vi "Open TCP Session.vi"(7 "Slave ID (255)":u8=255, 8 "error in (no error)":errorcluster, 9 "Timeout (10000)":i32=10000, 10 "Port (502)":u16=502, 11 "IP Address":string="localhost") -> (0 "error out":errorcluster, 3 "MB_TCP session":refnum<class "MB_Master_TCP.lvclass">)   [LabVIEW 2016, in "MB Master.lvlib" / "MB_Master_TCP.lvclass"]
doc: "Opens a new modbus session and establish the TCP connection. Note that the slave ID is set to the default of 0xFF. Slave ID can be changed later via the property node \"Slave ID\"."
uses:
  MB_Master_TCP.lvclass
  MB_ADU/MB_ADU.lvclass/MB_ADU.ctl
  MB_ADU_TCP/MB_ADU_TCP.lvclass/MB_ADU_TCP.ctl
  MB_Master_TCP.lvclass/MB_Master_TCP.ctl
  MB_ADU/Build ADU.vi
  MB_ADU_TCP/MB_ADU_TCP.lvclass
  C:/Users/PRANAV/Downloads/Modbus-Master-master (7)/Modbus-Master-master/MB_ADU/MB_ADU.lvclass
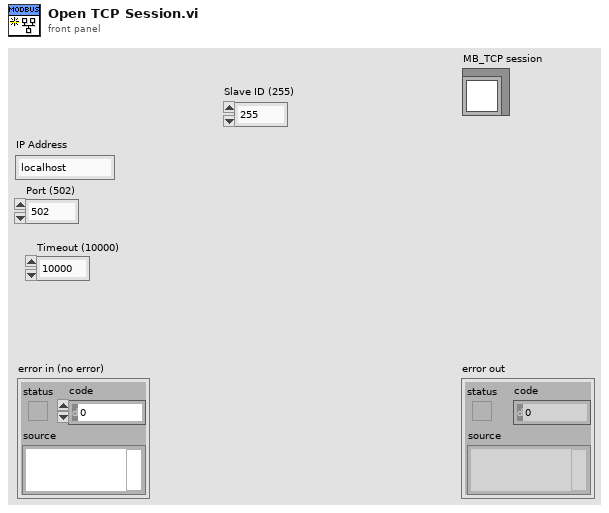
[diagram p1: front panel]
types:
  T1 = cluster{"IP Address":string, "Port":u16, "Timeout":i32, "Notifier":refnum<notifier>}
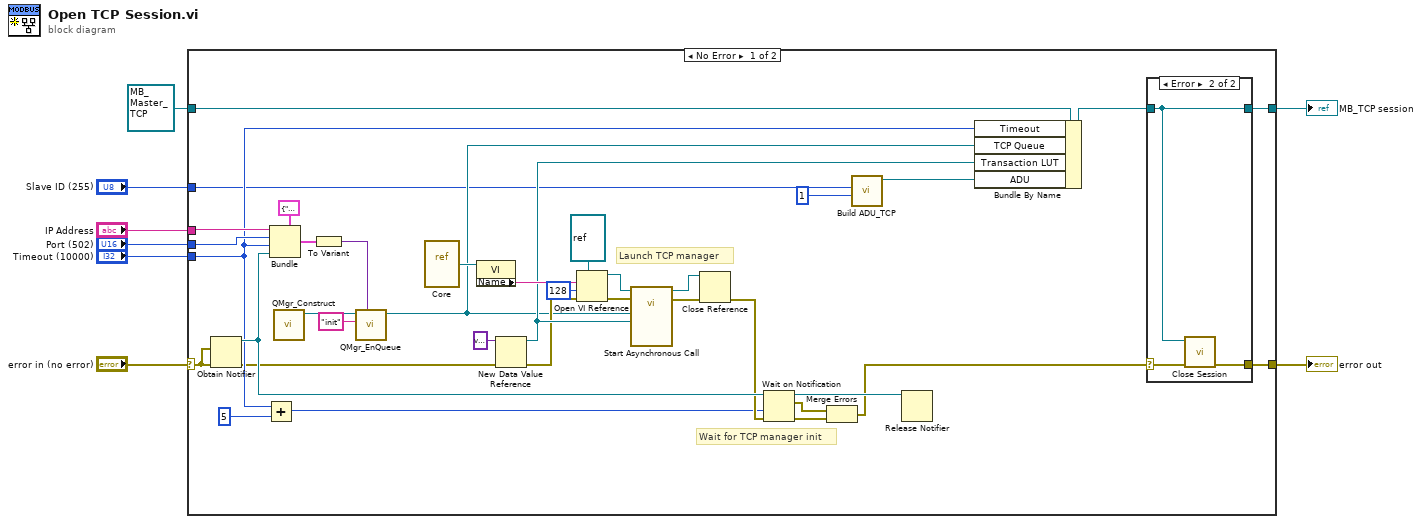
[diagram p0: block diagram]
diagram:
  n1 = case shown="No Error" "error in (no error)" {
    selector: "error in (no error)" -> [w22 w52]
    tunnel: [w26 w52] -> w7
    tunnel: [w28 w51] -> w5
    tunnel: refnum<class "MB_Master_TCP.lvclass"> refnum ("MB_Master_TCP in") -> [w45 w51]
    tunnel: "IP Address" -> [w41 _]
    tunnel: "Port (502)" -> [w40 _]
    tunnel: "Timeout (10000)" -> [w18 _]
    tunnel: "Slave ID (255)" -> [w9 _]
    frame No Error {
      # "Wait for TCP manager init"
      # "Launch TCP manager"
      n2 = Obtain Notifier(notification data type=w22, error in (no error)=w22) -> (notifier out=w31:refnum<notifier>, error out=w10:errorcluster)  [unwired: 2 in, 1 out]
      n3 = Add(x=w18, y=5) -> (x+y=w16:i32)
      n4 = Bundle(cluster=T1 {"IP Address"="", "Port"=502, "Timeout"=10000, "Notifier"=refnum}, "IP Address"=w41, "Port"=w40, "Timeout"=w18, "Notifier"=w31) -> (w33:T1)
      n5 = call "QMgr_Construct.vi"() -> ("queue out"=w14:refnum<queue>)  [unwired: 11 in]
      n6 = To Variant(anything=w33) -> (Variant=w12:variant)
      n7 = call "QMgr_EnQueue.vi"("Data"=w12, "Command"="init" ("cmd"), "queue in"=w14) -> ("queue out"=w11:refnum<queue>)  [unwired: 8 in]
      n8 = vi-ref "Core.vi"() -> (w35:refnum<vi>)
      n9 = property class="VI"(reference=w35) -> ("Name"=w36:string)  [unwired: 1 in, 2 out]
      n10 = New Data Value Reference(data value=variant ("variant"), error in=w10) -> (data value reference=w32:refnum<data-value>, error out=w21:errorcluster)
      n11 = Open VI Reference(type specifier VI Refnum (for type only)=refnum<vi> refnum, vi path=w36, options=128, error in (no error)=w21) -> (vi reference=w39:refnum<vi>, error out=w20:errorcluster)  [unwired: 2 in]
      n12 = call-by-ref "Start Asynchronous Call"(reference=w39, error in=w20, "Transaction LUT"=w32, "CMD Queue"=w11) -> (reference out=w25:refnum<vi>, error out=w24:errorcluster)  [unwired: 10 in]
      n13 = Close Reference(reference=w25, error in (no error)=w24) -> (error out=w23:errorcluster)
      n14 = Wait on Notification(notifier=w31, timeout in ms (-1)=w16, error in (no error)=w23) -> (notifier out=w19:refnum<notifier>, notification=w29:errorcluster, error out=w30:errorcluster)  [unwired: 1 in, 1 out]
      n15 = Merge Errors(w29, w30) -> (w15:errorcluster)
      n16 = call "Build ADU_TCP.vi"("Transaction ID"=u16 1, "Slave ID"=w9) -> ("MB_ADU_TCP out"=w44:refnum<class "MB_ADU_TCP.lvclass">)  [unwired: 8 in, 1 out]
      n17 = Release Notifier(notifier=w19) -> ()  [unwired: 2 in, 3 out]
      n18 = Bundle By Name(cluster=w45, "Timeout"=w18, "TCP Queue"=w11, "Transaction LUT"=w32, "ADU"=w44) -> (w27:refnum<class "MB_Master_TCP.lvclass">)
      n19 = case shown="Error" w15 {
        selector: w15 -> [w46 w48]
        tunnel: [w47 w49] -> w28
        tunnel: w27 -> [w47 w49]
        tunnel: [w46 w50] -> w26
        frame No Error {
        }
        frame Error {
          n20 = call-dynamic "Close Session.vi"("error in (no error)"=w48, "MB TCP session"=w49) -> ("error out"=w50:errorcluster)  [unwired: 9 in]
        }
      }
    }
    frame Error {
    }
  }
  "error out" <- w7
  "MB_TCP session" <- w5
